vi "get_token_type.vi"(11 "token":string) -> (3 "ExpressionType":T1)   [LabVIEW 2020]
uses:
  ExpressionType.ctl
  <vilib>/regexp/Match Regular Expression.xnode
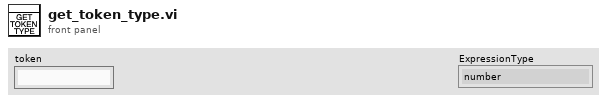
[diagram p1: front panel]
types:
  T1 = typedef "ExpressionType.ctl" = enum16{"number", "string", "symbol", "primitive", "list", "closure", "macro", "nil", "error"}
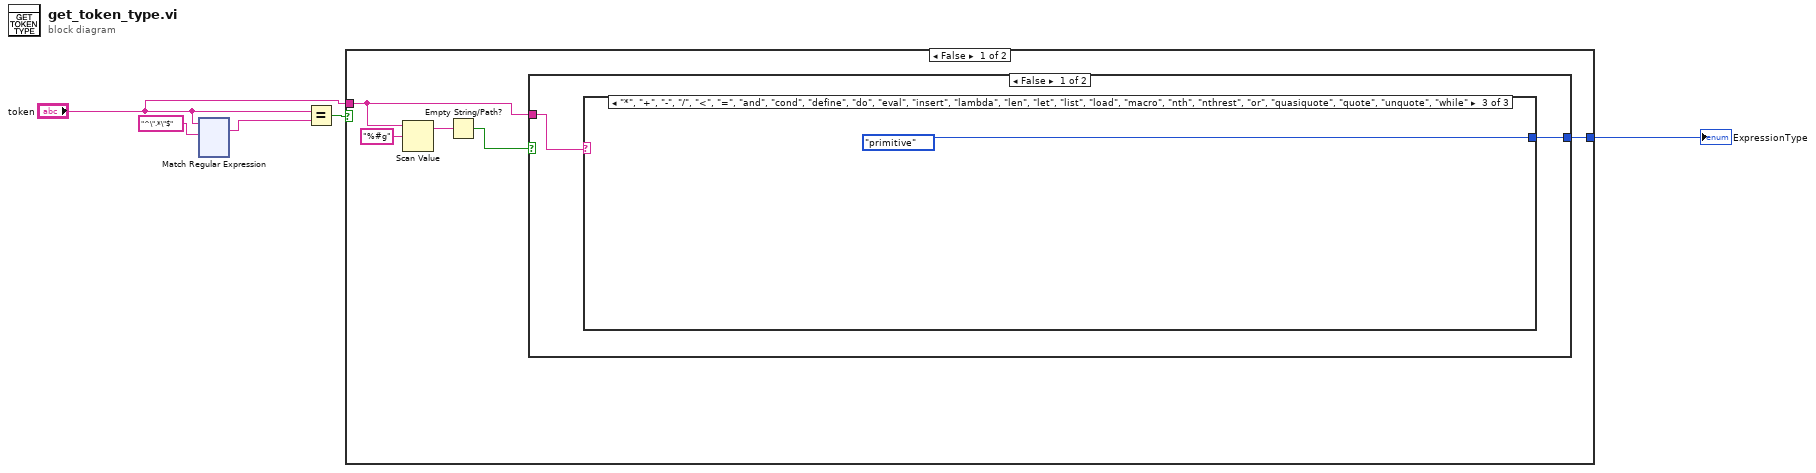
[diagram p0: block diagram]
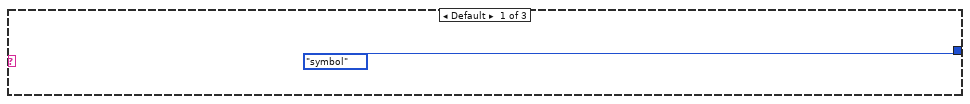
[diagram p2: hidden frame]
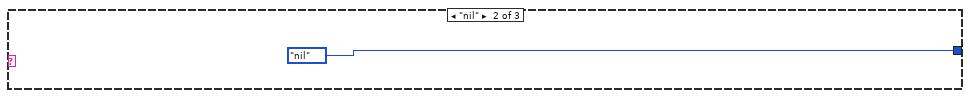
[diagram p3: hidden frame]
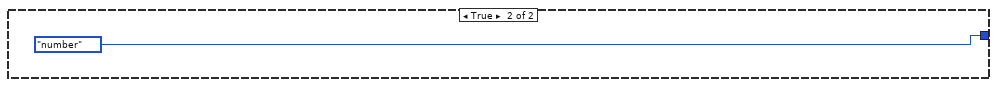
[diagram p4: hidden frame]
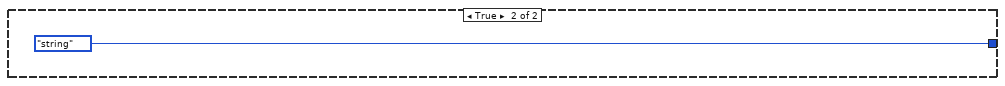
[diagram p5: hidden frame]
diagram:
  n1 = xnode "Match Regular Expression"("input string"="token", "regular expression"="^\".*\"$") -> ("whole match"=w1:string)  [unwired: 4 in, 4 out]
  n2 = Equal?(x="token", y=w1) -> (x = y?=w3:bool)
  n3 = case shown="False" w3 {
    tunnel: "token" -> [w9 _]
    tunnel: [w10 ExpressionType."string" ("ExpressionType")] -> w4
    frame False {
      n4 = Scan Value(string=w9, format string="%#g") -> (output string=w7:string)  [unwired: 1 in, 1 out]
      n5 = Empty String/Path?(string/path=w7) -> (empty?=w6:bool)
      n6 = case shown="False" w6 {
        tunnel: [w12 ExpressionType."number" ("ExpressionType")] -> w10
        tunnel: w9 -> [w11 _]
        frame False {
          n7 = case shown="\"*\", \"+\", \"-\", \"/\", \"<\", \"=\", \"and\", \"cond\", \"define\", \"do\", \"eval\", \"insert\", \"lambda\", \"len\", \"let\", \"list\", \"load\", \"macro\", \"nth\", \"nthrest\", \"or\", \"quasiquote\", \"quote\", \"unquote\", \"while\"" w11 {
            tunnel: [ExpressionType."symbol" ("ExpressionType") ExpressionType."nil" ("ExpressionType") ExpressionType."primitive" ("ExpressionType")] -> w12
            frame Default {
            }
            frame "nil" {
            }
            frame "*", "+", "-", "/", "<", "=", "and", "cond", "define", "do", "eval", "insert", "lambda", "len", "let", "list", "load", "macro", "nth", "nthrest", "or", "quasiquote", "quote", "unquote", "while" {
            }
          }
        }
        frame True {
        }
      }
    }
    frame True {
    }
  }
  "ExpressionType" <- w4
